vi "simpleInterpreter3.vi"() -> ()   [LabVIEW 2011]
uses:
  <vilib>/Utility/inputDevices.llb/keyboardAcquire.vi
  kernel32.dll
  systemlib/labviewwait.dll
panel:
  out "lua_type":i32(ring) items=["LUA_TNONE"=-1, "LUA_TNIL"=0, "LUA_TBOOLEAN"=1, "LUA_TLIGHTUSERDATA"=2, "LUA_TNUMBER "=3, "LUA_TSTRING"=4, "LUA_TTABLE"=5, "LUA_TFUNCTION"=6, "LUA_TUSERDATA"=7, "LUA_TTHREAD"=8, "LUA_NUMTAGS "=9]
  out "lua_State *commandthread":u64
  out "lua_State *L":u64
  out "lua_State *print thread":u64
  in  "status refrash":bool
  in  "command refrash":bool
  out "stack":i32
  out "LoadBufferStatus":i32(ring) items=["LUA_OK", "LUA_YIELD", "LUA_ERRRUN", "LUA_ERRSYNTAX", "LUA_ERRMEM", "LUA_ERRGCMM", "LUA_ERRERR"]
  out "PcallStatus":i32(ring) items=["LUA_OK", "LUA_YIELD", "LUA_ERRRUN", "LUA_ERRSYNTAX", "LUA_ERRMEM", "LUA_ERRGCMM", "LUA_ERRERR"]
  in  "停止":bool
  in  "command(ctrl+enter)":string
  out "status":string
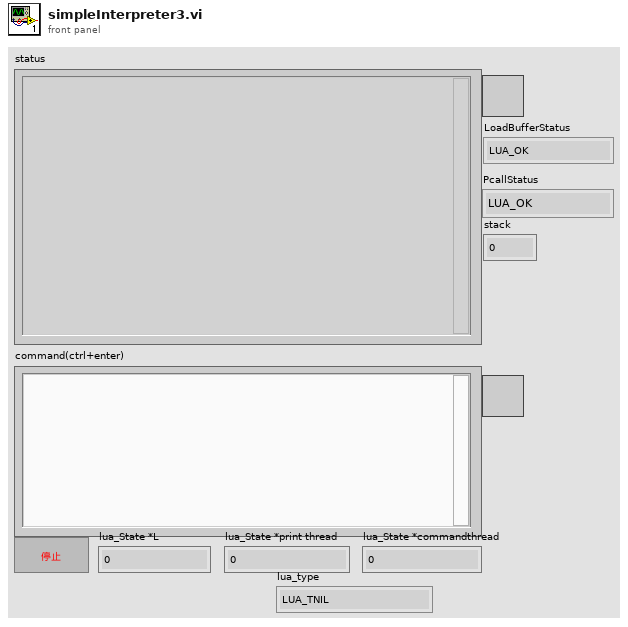
[diagram p1: front panel]
types:
  T1 = enum16{"0", "1", "2", "3", "4", "5", "6", "7", "8", "9", "A", "B", "C", "D", "E", "F", "G", "H", "I", "J", "K", "L", "M", "N", "O", "P", "Q", "R", "S", "T", "U", "V", "W", "X", "Y", "Z", "F1", "F2", "F3", "F4", "F5", "F6", "F7", "F8", "F9", "F10", "F11", "F12", "F13", "F14", "F15", "ADD", "BACK", "BACKSLASH", "CAPITAL", "COMMA", "DECIMAL", "DELETE", "DIVIDE", "DOWN", "END", "EQUALS", "ESCAPE", "GRAVE (`)", "HOME", "INSERT", "LBRACKET", "LCONTROL", "LEFT", "L ALT", "LSHIFT", "LWIN", "MINUS", "MULTIPLY", "NEXT", "NUMLOCK", "NUMPAD_0", "NUMPAD_1", "NUMPAD_2", "NUMPAD_3", "NUMPAD_4", "NUMPAD_5", "NUMPAD_6", "NUMPAD_7", "NUMPAD_8", "NUMPAD_9", "PAUSE", "PERIOD", "PRIOR (PG UP)", "RBRACKET", "RCONTROL", "RETURN", "RIGHT", "R ALT", "RSHIFT", "RWIN", "SCROLL", "SEMICOLON", "SLASH", "SPACE", "SUBTRACT", "TAB", "UP", "ENTER (num pad)", "' (quote)"}[]
  T2 = enum16{"0", "1", "2", "3", "4", "5", "6", "7", "8", "9", "A", "B", "C", "D", "E", "F", "G", "H", "I", "J", "K", "L", "M", "N", "O", "P", "Q", "R", "S", "T", "U", "V", "W", "X", "Y", "Z", "F1", "F2", "F3", "F4", "F5", "F6", "F7", "F8", "F9", "F10", "F11", "F12", "F13", "F14", "F15", "ADD", "BACK", "BACKSLASH", "CAPITAL", "COMMA", "DECIMAL", "DELETE", "DIVIDE", "DOWN", "END", "EQUALS", "ESCAPE", "GRAVE (`)", "HOME", "INSERT", "LBRACKET", "LCONTROL", "LEFT", "L ALT", "LSHIFT", "LWIN", "MINUS", "MULTIPLY", "NEXT", "NUMLOCK", "NUMPAD_0", "NUMPAD_1", "NUMPAD_2", "NUMPAD_3", "NUMPAD_4", "NUMPAD_5", "NUMPAD_6", "NUMPAD_7", "NUMPAD_8", "NUMPAD_9", "PAUSE", "PERIOD", "PRIOR (PG UP)", "RBRACKET", "RCONTROL", "RETURN", "RIGHT", "R ALT", "RSHIFT", "RWIN", "SCROLL", "SEMICOLON", "SLASH", "SPACE", "SUBTRACT", "TAB", "UP", "ENTER (num pad)", "' (quote)"}
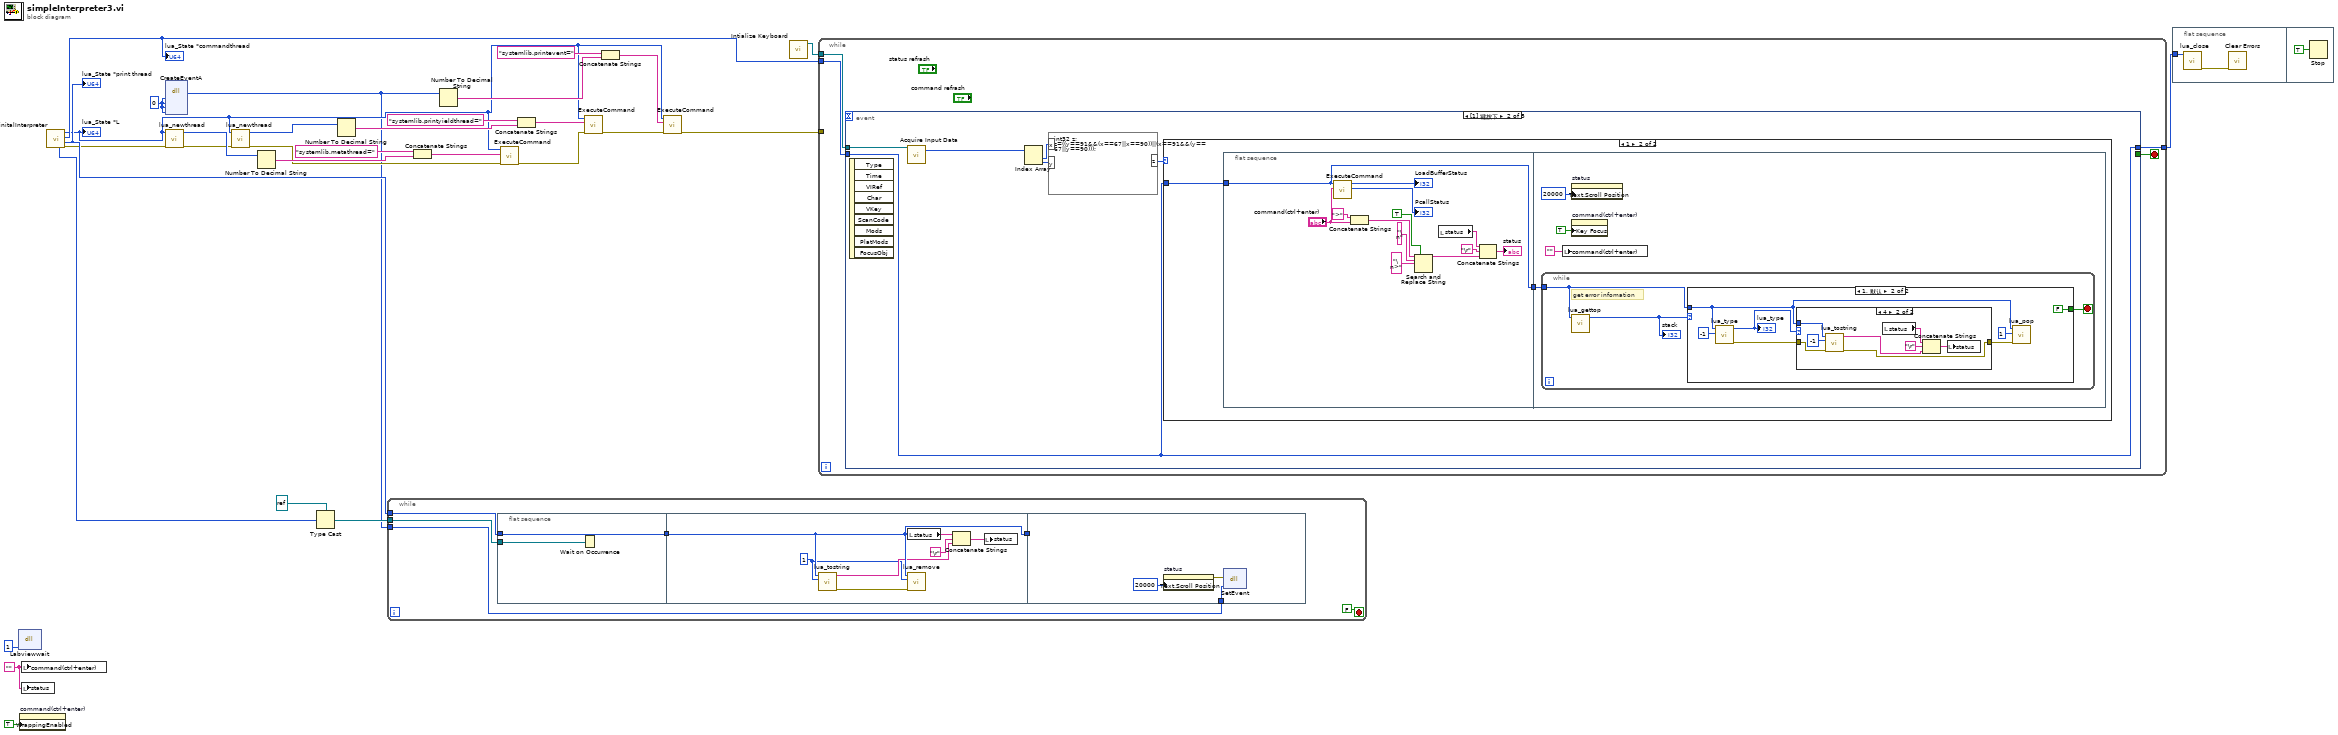
[diagram p0: block diagram]
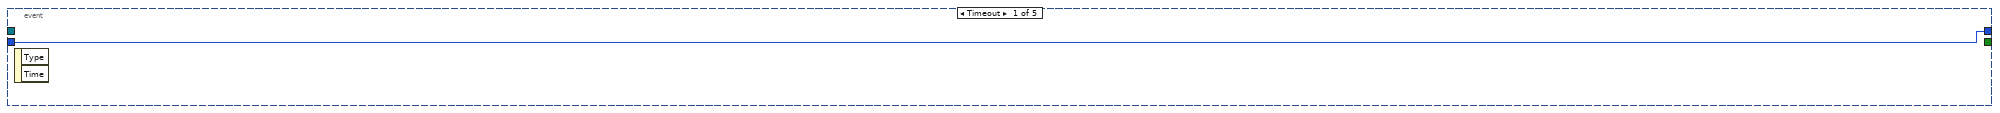
[diagram p2: hidden frame]
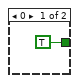
[diagram p4: hidden frame]
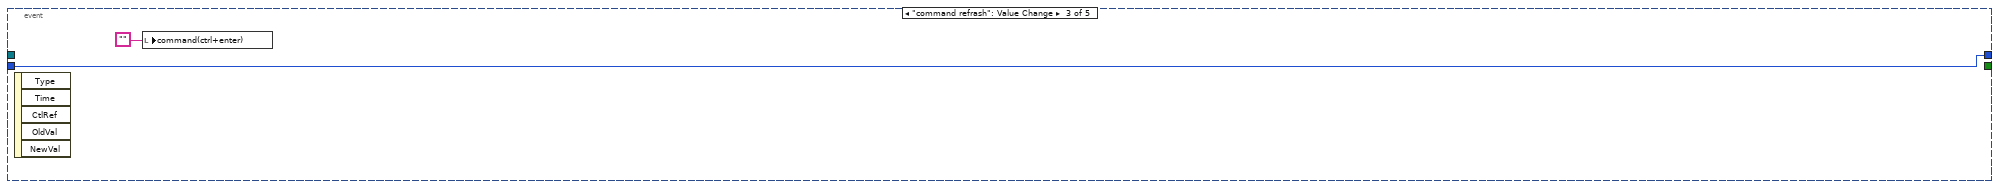
[diagram p6: hidden frame]
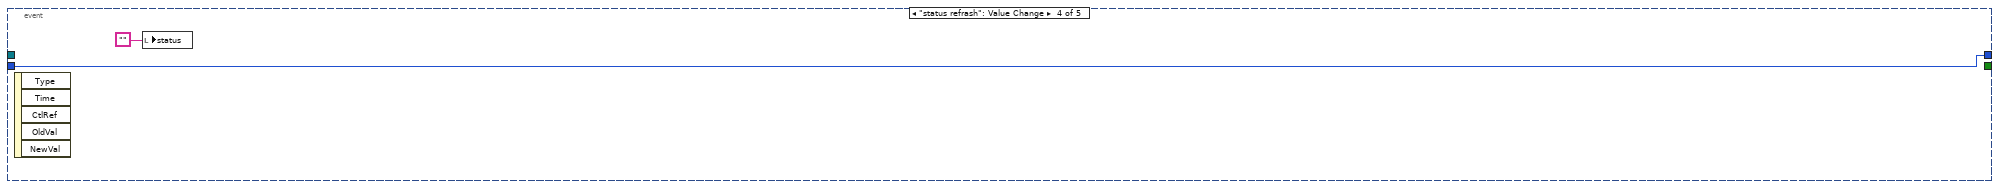
[diagram p7: hidden frame]
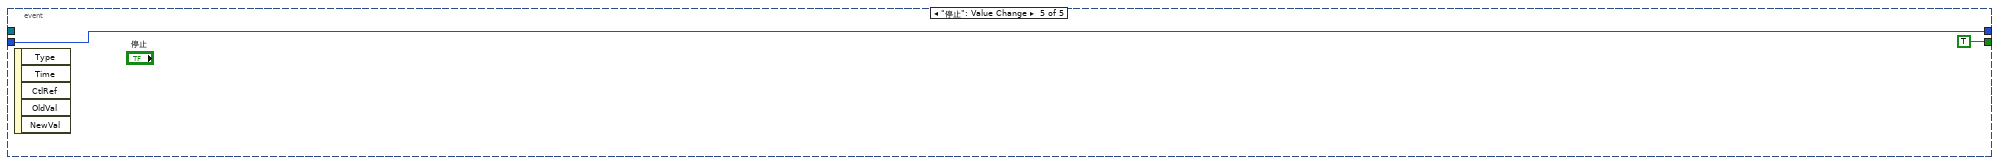
[diagram p8: hidden frame]
diagram:
  w2 = i8 0 ("LPSECURITY_ATTRIBUTES lpEventAttributes")
  w30 = ""
  n1 = dll-call lib="G:/My DBank/_work_pan/monkey task 2012/systemlib/labviewwait.dll" fn="Labviewwait"("wait"=1) -> ()  [unwired: 5 in, 2 out]
  n2 = property on="command(ctrl+enter)" class="Str"("WrappingEnabled"=TRUE ("启用自动换行")) -> ()  [unwired: 2 in, 2 out]
  n3 = local write "command(ctrl+enter)"(w30) -> ()
  n4 = local write "status"(w30) -> ()
  n5 = call "initalInterpreter.vi"() -> ("错误输出"=w16:errorcluster, "lua_State *print thread"=w23:u64, "lua_State *commandthread"=w10:u64, "lua_State *mainthread"=w3:u64, "printoccur"=w24:i32)  [unwired: 5 in, 2 out]
  "lua_State *print thread" <- w23
  "lua_State *L" <- w3
  "lua_State *commandthread" <- w10
  n6 = dll-call lib="kernel32.dll" fn="CreateEventA"("LPSECURITY_ATTRIBUTES lpEventAttributes"=w2, "BOOL bManualReset"=w2, "BOOL bInitialState"=w2, "LPCTSTR lpName"=w2) -> ("HANDLE CreateEvent"=w1:i32)  [unwired: 7 in, 2 out]
  n7 = call "lua_newthread.vi"("error in"=w16, "lua_State *L"=w3) -> ("error out"=w15:errorcluster, "lua_State *lua_newthread"=w20:u64)  [unwired: 8 in]
  n8 = call "lua_newthread.vi"("error in"=w15, "lua_State *L"=w3) -> ("error out"=w14:errorcluster, "lua_State *lua_newthread"=w11:u64)  [unwired: 8 in]
  n9 = Number To Decimal String(number=w20) -> (decimal integer string=w22:string)  [unwired: 1 in]
  n10 = Type Cast(type=refnum<k4> refnum ("事件发生"), x=w24) -> (*(type *) &x=w25:refnum<k4>)
  n11 = Number To Decimal String(number=w11) -> (decimal integer string=w13:string)  [unwired: 1 in]
  n12 = while {
    tunnel: w23 -> [w35]
    tunnel: w25 -> [w32]
    tunnel: w1 -> [w31]
    stop <- FALSE stop-if-true
    n13 = flat-sequence {
      tunnel: w35 -> [w38]
      tunnel: [w38] -> w33
      tunnel: w32 -> [w37]
      tunnel: [w45] -> w34
      tunnel: w33 -> [w45]
      tunnel: w34 -> [_]
      tunnel: w31 -> [w46]
      frame #0 {
        n14 = Wait on Occurrence(2:w37) -> ()  [unwired: 2 in, 1 out]
      }
      frame #1 {
        w39 = 1 ("index")
        n15 = call "lua_tostring.vi"("index"=w39, "lua_State *L"=w45) -> ("error out"=w40:errorcluster, "constant string"=w41:string)  [unwired: 8 in]
        n16 = local read "status"() -> (w43:string)
        n17 = call "lua_remove.vi"("error in"=w40, "int index"=w39, "lua_State *L"=w45) -> ()  [unwired: 8 in, 1 out]
        n18 = Concatenate Strings(w43, "\r", w41) -> (w44:string)
        n19 = local write "status"(w44) -> ()
      }
      frame #2 {
        n20 = property on="status" class="Str"("Text.Scroll Position"=u32 20000 ("文本.滚动条位置")) -> (error out=w47:errorcluster)  [unwired: 2 in, 1 out]
        n21 = dll-call lib="kernel32.dll" fn="SetEvent"(error in=w47, "参数1"=w46) -> ()  [unwired: 4 in, 2 out]
      }
    }
  }
  n22 = Concatenate Strings("systemlib.metathread=" ("字符串"), w22) -> (w19:string)
  n23 = Number To Decimal String(number=w1) -> (decimal integer string=w8:string)  [unwired: 1 in]
  n24 = call "ExecuteCommand.vi"("error in"=w14, "command(ctrl+enter)"=w19, "lua_State *luaL_newstate"=w3) -> ("error out"=w18:errorcluster)  [unwired: 6 in, 2 out]
  n25 = Concatenate Strings("systemlib.printyieldthread=" ("字符串"), w13) -> (w12:string)
  n26 = call "ExecuteCommand.vi"("error in"=w18, "command(ctrl+enter)"=w12, "lua_State *luaL_newstate"=w3) -> ("error out"=w4:errorcluster)  [unwired: 6 in, 2 out]
  n27 = Concatenate Strings("systemlib.printevent=" ("字符串"), w8) -> (w6:string)
  n28 = call "ExecuteCommand.vi"("error in"=w4, "command(ctrl+enter)"=w6, "lua_State *luaL_newstate"=w3) -> ("error out"=w5:errorcluster)  [unwired: 6 in, 2 out]
  n29 = call <vilib>:"Intialize Keyboard.vi"() -> ("device ID"=w28:refnum<k1>)  [unwired: 10 in, 1 out]
  n30 = while {
    tunnel: w10 -> [w52]
    tunnel: [w50] -> w27
    tunnel: w28 -> [w49]
    tunnel: w5 -> [_]
    stop <- w51 stop-if-true
    n31 = event shown="[1] 键按下" {
      selector: _ -> [_ _ _ _ _]
      dyn-events: _ -> [_ _ _ _ _]
      timeout: _ -> [_ _ _ _ _]
      tunnel: w52 -> [w53 w54 w99 w101 w103]
      tunnel: [_ _ _ _ TRUE ("停止 2")] -> w51
      tunnel: [w53 w54 w99 w101 w103] -> w50
      tunnel: w49 -> [_ w59 _ _ _]
      event Timeout {
        n32 = event-data() -> ()  [unwired: 1 in, 2 out]
      }
      event Key Down {
        n33 = event-data() -> ()  [unwired: 1 in, 9 out]
        n34 = call-poly <vilib>:"Acquire Input Data.vi"("device ID"=w59) -> ("keys pressed"=w58:T1)  [unwired: 16 in, 2 out]
        n35 = Index Array(array=w58) -> (element #1=w57:T2, element #2=w56:T2)  [unwired: 2 in]
        n36 = formula code="int32 z;\nz=((y==91&&(x==67||x==90))||(x==91&&(y==67||y==90)));"("x"=w57, "y"=w56) -> ("z"=w55:i32)
        n37 = case shown="1" w55 {
          tunnel: w54 -> [_ w61]
          frame 0, Default {
          }
          frame 1 {
            n38 = flat-sequence {
              tunnel: w61 -> [w62]
              tunnel: [w62] -> w60
              tunnel: w60 -> [w75]
              frame #0 {
                n39 = call "ExecuteCommand.vi"("command(ctrl+enter)"="command(ctrl+enter)", "lua_State *luaL_newstate"=w62) -> ("thread status 2"=→"PcallStatus":i32, "thread status"=→"LoadBufferStatus":i32)  [unwired: 7 in, 1 out]
                n40 = Concatenate Strings(">", "command(ctrl+enter)") -> (w67:string)
                n41 = Search and Replace String(replace all?=TRUE ("替换全部？(F)"), input string=w67, search string="\n" ("搜索字符串"), replace string="\n>" ("替换字符串(\"\")")) -> (result string=w63:string)  [unwired: 4 in, 3 out]
                n42 = local read "status"() -> (w73:string)
                n43 = Concatenate Strings(w73, "\r", w63) -> (→"status":string)
              }
              frame #1 {
                n44 = while {
                  tunnel: w75 -> [w80]
                  stop <- w79 stop-if-true
                  # "get error infomation"
                  n45 = call "lua_gettop.vi"("lua_State *L"=w80) -> ("lua_gettop"=w81:i32)  [unwired: 9 in, 1 out]
                  "stack" <- w81
                  n46 = case shown="1, 默认" w81 {
                    tunnel: w80 -> [_ w86]
                    tunnel: [TRUE FALSE] -> w79
                    frame 0 {
                    }
                    frame 1, Default {
                      n47 = call "lua_type.vi"("int index"=-1, "lua_State *L"=w86) -> ("error out"=w88:errorcluster, "lua_type"=w83:i32)  [unwired: 8 in]
                      "lua_type" <- w83
                      n48 = case shown="4" w83 {
                        tunnel: w88 -> [w90 w98]
                        tunnel: [w90 w97] -> w87
                        tunnel: w86 -> [_ w96]
                        frame 0, Default {
                        }
                        frame 4 {
                          n49 = call "lua_tostring.vi"("error in"=w98, "index"=-1, "lua_State *L"=w96) -> ("error out"=w97:errorcluster, "constant string"=w91:string)  [unwired: 7 in]
                          n50 = local read "status"() -> (w93:string)
                          n51 = Concatenate Strings(w93, "\r", w91) -> (w92:string)
                          n52 = local write "status"(w92) -> ()
                        }
                      }
                      n53 = call "lua_pop.vi"("error in"=w87, "n"=1, "lua_State *L"=w86) -> ()  [unwired: 8 in, 1 out]
                    }
                  }
                }
                n54 = local write "command(ctrl+enter)"("") -> ()
                n55 = property on="status" class="Str"("Text.Scroll Position"=u32 20000 ("文本.滚动条位置")) -> ()  [unwired: 2 in, 2 out]
                n56 = property on="command(ctrl+enter)" class="Str"("Key Focus"=TRUE ("键选中")) -> ()  [unwired: 2 in, 2 out]
              }
            }
          }
        }
      }
      event "command refrash": Value Change {
        n57 = event-data() -> ()  [unwired: 1 in, 5 out]
        n58 = local write "command(ctrl+enter)"("") -> ()
      }
      event "status refrash": Value Change {
        n59 = event-data() -> ()  [unwired: 1 in, 5 out]
        n60 = local write "status"("") -> ()
      }
      event "停止": Value Change {
        n61 = event-data() -> ()  [unwired: 1 in, 5 out]
      }
    }
  }
  n62 = flat-sequence {
    tunnel: w27 -> [w106]
    frame #0 {
      n63 = call "lua_close.vi"("lua_State *L"=w106) -> ("error out"=w105:errorcluster)  [unwired: 10 in]
      n64 = call <vilib>:"Clear Errors.vi"("error in (no error)"=w105) -> ()  [unwired: 6 in, 1 out]
    }
    frame #1 {
      n65 = Stop(stop? (T)=TRUE ("停止？(T)")) -> ()
    }
  }
